vi "Replace_Array_Subset_2D_SubArray_Rows.vi"(9 "SubArray RAS2D":i8[](array[numeric]), 10 "Index Row":i32, 11 "RAS2D":i8[][](array[numeric])) -> (3 "New Array RAS2D":i8[][](array[numeric]))   [LabVIEW 2018]
panel:
  out "Size":i32
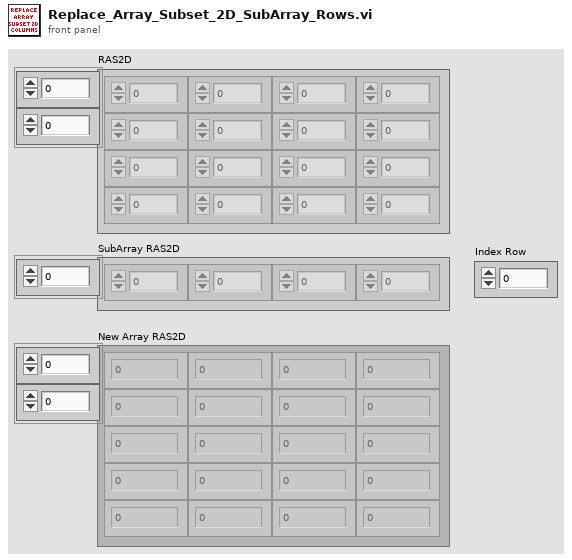
[diagram p1: front panel]
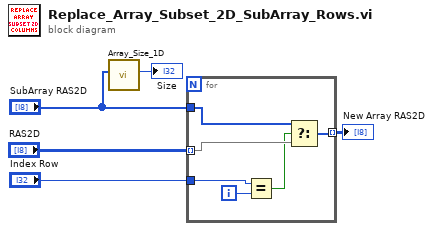
[diagram p0: block diagram]
diagram:
  n1 = call "Array_Size_1D.vi"("Array"="SubArray RAS2D") -> ("Size"=→"Size":i32)  [unwired: 10 in]
  n2 = for {
    tunnel: "RAS2D" -> [w11] mode=indexing
    tunnel: [w10] -> w2 mode=indexing
    tunnel: "SubArray RAS2D" -> [w8]
    tunnel: "Index Row" -> [w6]
    i -> [w9]
    n3 = Equal?(x=w6, y=w9) -> (x = y?=w7:bool)
    n4 = Select(t=w8, s=w7, f=w11) -> (s? t:f=w10:i8[])
  }
  "New Array RAS2D" <- w2
